vi "GetChannel.vi"(7 "Name":string, 11 "Channels":T1[](array[typedef])) -> (3 "Channel":T1, 5 "Found?":bool)   [LabVIEW 2014, in "DigitizerPlugins.lvlib" / "DigitizerBase.lvclass"]
uses:
  DigitizerBase.lvclass
  Typedefs/Channel.ctl
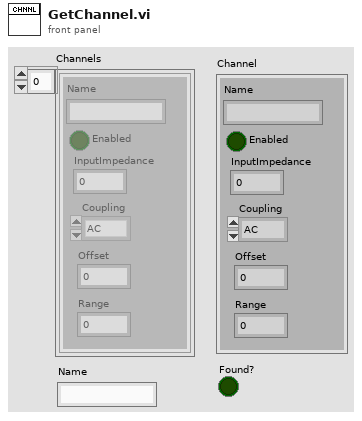
[diagram p1: front panel]
types:
  T1 = typedef "DigitizerPlugins.lvlib/DigitizerBase.lvclass/Channel.ctl" = cluster{"Name":string, "Enabled":bool, "InputImpedance":dbl, "Coupling":enum16{"AC", "DC", "Gnd"}, "Offset":dbl, "Range":dbl}
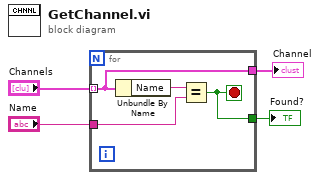
[diagram p0: block diagram]
diagram:
  n1 = for {
    tunnel: "Channels" -> [w6] mode=indexing
    tunnel: "Name" -> [w7]
    tunnel: [w6] -> w2
    tunnel: [w5] -> w1
    stop <- w5 stop-if-true
    n2 = Unbundle By Name(w6) -> ("Name"=w8:string)
    n3 = Equal?(x=w8, y=w7) -> (x = y?=w5:bool)
  }
  "Found?" <- w1
  "Channel" <- w2
